vi "Compute Pseudo USC v2.vi"(4 "SDV (s)":dbl=160.0, 6 "Gaussian IRF":bool, 8 "Error In":errorcluster, 10 "Phasor Parameters":T2={"Display Parameters"={"# Points"=0, "Ramp Type"=enum."Linear", "Type of Series"=enum."1-Exp Decays", "Min tau"=0.0, "Max tau"=0.0, "Include 0"=FALSE, "Include Infinity"=FALSE}, "Phasor Parameters"={"Harmonic frequency"=0.0, "Use f* = 1/D Frequency"=FALSE, "Calibrated Phasor"=FALSE, "Calibration Lifetime"=1e-09, "Phasor Calculation"=enum."Direct Sum", "SEPL Type"=enum."UC", "# Gates"=1.0, "Square Gate Width"=1e-09, "Show Ticks"=FALSE}, "Decay & IRF Parameters"={"Lifetime"=0.0, "IRF Offset"=0.0, "Laser Period"=0.0, "Normalized Decays"=FALSE, "IRF Model"=enum."Dirac", "IRF Parameter 1"=0.0}, "Gate Parameters"={"First Gate Start"=0.0, "Use Gate Center"=FALSE, "Gate Width"=0.0, "Gate Step"=0.0, "# Gates"=0.0, "Gate Type"=enum."Square", "Edge Width"=0.0, "Top Slope"=0.0, "Reversed Sawtooth?"=FALSE, "Analytical Computation"=FALSE, "Tolerance"=1.0, "Integration"=enum."Item 0", "# Steps"=1.0, "Type of User-defined Function"=enum."Gate"}, "Detector Parameters"={"Frames/Image"=0, "Gates/Frame"=0, "Bits/Frame"=0, "Multiplicity"=0, "Incident Signal"=0.0}} {"Detector Parameters"."Frames/Image" min=1; "Detector Parameters"."Multiplicity" min=0; "Detector Parameters"."Bits/Frame" min=1; "Detector Parameters"."Gates/Frame" min=1; "Gate Parameters"."# Steps" min=0.0; "Gate Parameters"."Tolerance" min=0.0; "Gate Parameters"."Top Slope" min=0.0; "Gate Parameters"."Edge Width" min=0.0; "Gate Parameters"."Gate Step" min=0.0; "Gate Parameters"."# Gates" min=0.0 step=1.0; "Gate Parameters"."Gate Width" min=0.0; "Decay & IRF Parameters"."Lifetime" min=0.0; "Decay & IRF Parameters"."Laser Period" min=0.0; "Phasor Parameters"."Square Gate Width" min=0.0; "Phasor Parameters"."# Gates" min=0.0; "Phasor Parameters"."Calibration Lifetime" min=0.0; "Phasor Parameters"."Harmonic frequency" min=0.0; "Display Parameters"."Min tau" min=0.0; "Display Parameters"."Max tau" min=0.0; "Display Parameters"."# Points" min=1 step=1}, 11 "Phasor Graph Refnum":refnum<vi>) -> (0 "Error Out":errorcluster, 1 "Plot Name":string, 2 "Lifetime/Fraction Array":dbl[](array[numeric]), 3 "Single Exponential Phasor Plot":cluster{"Array":dbl[], "Array":dbl[]}, 5 "Phasor Calculation":T6, 7 "CPU (s)":dbl)   [LabVIEW 2019]
uses:
  Pseudo Phasor Parameters.ctl
  Phasor Explorer Display Parameters.ctl
  Type of Series.ctl
  Phasor Explorer Phasor Parameters.ctl
  Phasor Calculation Type.ctl
  Phasor Type.ctl
  Phasor Explorer Decay Parameters.ctl
  IRF Model.ctl
  Phasor Explorer Gate Parameters.ctl
  Gate Type.ctl
  Phasor Explorer Detector Parameters.ctl
  SEPXP Phasor Plot Info.ctl
  Phasor Calibration Data.ctl
  Phasor UC_N[W] Parameters.ctl
  <vilib>/Utility/High Resolution Relative Seconds.vi
panel:
  out "Plot Metadata":T1={"Lifetime/Fraction Array"=[], "Phasor Explorer Parameters"={"Display Parameters"={"# Points"=0, "Ramp Type"=enum."Linear", "Type of Series"=enum."1-Exp Decays", "Min tau"=0.0, "Max tau"=0.0, "Include 0"=FALSE, "Include Infinity"=FALSE}, "Phasor Parameters"={"Harmonic frequency"=0.0, "Use f* = 1/D Frequency"=FALSE, "Calibrated Phasor"=FALSE, "Calibration Lifetime"=1e-09, "Phasor Calculation"=enum."Direct Sum", "SEPL Type"=enum."UC", "# Gates"=1.0, "Square Gate Width"=1e-09, "Show Ticks"=FALSE}, "Decay & IRF Parameters"={"Lifetime"=0.0, "IRF Offset"=0.0, "Laser Period"=0.0, "Normalized Decays"=FALSE, "IRF Model"=enum."Dirac", "IRF Parameter 1"=0.0}, "Gate Parameters"={"First Gate Start"=0.0, "Use Gate Center"=FALSE, "Gate Width"=0.0, "Gate Step"=0.0, "# Gates"=0.0, "Gate Type"=enum."Square", "Edge Width"=0.0, "Top Slope"=0.0, "Reversed Sawtooth?"=FALSE, "Analytical Computation"=FALSE, "Tolerance"=1.0, "Integration"=enum."Item 0", "# Steps"=1.0, "Type of User-defined Function"=enum."Gate"}, "Detector Parameters"={"Frames/Image"=0, "Gates/Frame"=0, "Bits/Frame"=0, "Multiplicity"=0, "Incident Signal"=0.0}}, "Phase Lifetimes"=[], "Modulus Lifetimes"=[]} {"Phasor Explorer Parameters"."Detector Parameters"."Frames/Image" min=1; "Phasor Explorer Parameters"."Detector Parameters"."Multiplicity" min=0; "Phasor Explorer Parameters"."Detector Parameters"."Bits/Frame" min=1; "Phasor Explorer Parameters"."Detector Parameters"."Gates/Frame" min=1; "Phasor Explorer Parameters"."Gate Parameters"."# Steps" min=0.0; "Phasor Explorer Parameters"."Gate Parameters"."Tolerance" min=0.0; "Phasor Explorer Parameters"."Gate Parameters"."Top Slope" min=0.0; "Phasor Explorer Parameters"."Gate Parameters"."Edge Width" min=0.0; "Phasor Explorer Parameters"."Gate Parameters"."Gate Step" min=0.0; "Phasor Explorer Parameters"."Gate Parameters"."# Gates" min=0.0 step=1.0; "Phasor Explorer Parameters"."Gate Parameters"."Gate Width" min=0.0; "Phasor Explorer Parameters"."Decay & IRF Parameters"."Lifetime" min=0.0; "Phasor Explorer Parameters"."Decay & IRF Parameters"."Laser Period" min=0.0; "Phasor Explorer Parameters"."Phasor Parameters"."Square Gate Width" min=0.0; "Phasor Explorer Parameters"."Phasor Parameters"."# Gates" min=0.0; "Phasor Explorer Parameters"."Phasor Parameters"."Calibration Lifetime" min=0.0; "Phasor Explorer Parameters"."Phasor Parameters"."Harmonic frequency" min=0.0; "Phasor Explorer Parameters"."Display Parameters"."Min tau" min=0.0; "Phasor Explorer Parameters"."Display Parameters"."Max tau" min=0.0; "Phasor Explorer Parameters"."Display Parameters"."# Points" min=1 step=1}
  out "# Rejected Pairs":i32
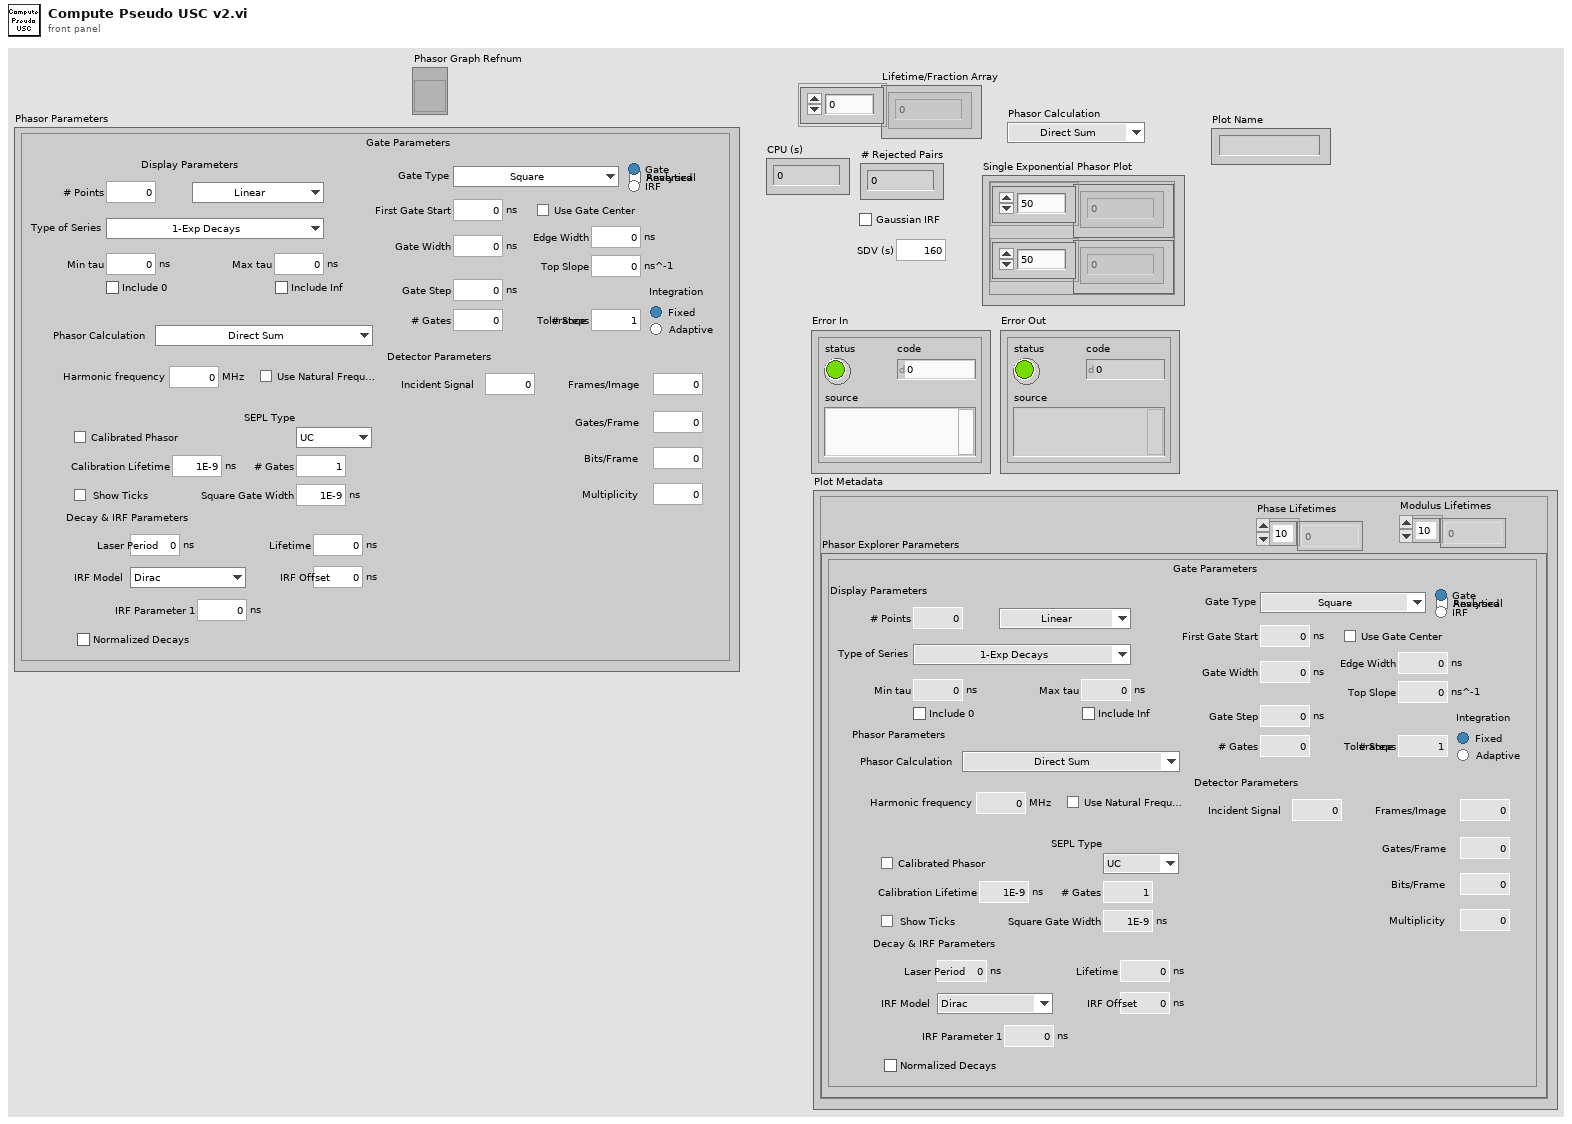
[diagram p1: front panel]
types:
  T1 = typedef "SEPXP Phasor Plot Info.ctl" = cluster{"Lifetime/Fraction Array":dbl[], "Phasor Explorer Parameters":T2, "Phase Lifetimes":dbl[], "Modulus Lifetimes":dbl[]}
  T2 = typedef "Pseudo Phasor Parameters.ctl" = cluster{"Display Parameters":T3, "Phasor Parameters":T5, "Decay & IRF Parameters":T8, "Gate Parameters":T10, "Detector Parameters":T12}
  T3 = typedef "Phasor Explorer Display Parameters.ctl" = cluster{"# Points":i32, "Ramp Type":enum16{"Linear", "Logarithmic"}, "Type of Series":T4, "Min tau":dbl[unit], "Max tau":dbl[unit], "Include 0":bool, "Include Infinity":bool}
  T4 = typedef "Type of Series.ctl" = enum16{"1-Exp Decays", "Linear Combination of 1-Exp"}
  T5 = typedef "Phasor Explorer Phasor Parameters.ctl" = cluster{"Harmonic frequency":dbl[unit], "Use f* = 1/D Frequency":bool, "Calibrated Phasor":bool, "Calibration Lifetime":dbl[unit], "Phasor Calculation":T6, "SEPL Type":T7, "# Gates":dbl, "Square Gate Width":dbl[unit], "Show Ticks":bool}
  T6 = typedef "Phasor Calculation Type.ctl" = enum16{"Direct Sum", "Analytical Formula"}
  T7 = typedef "Phasor Type.ctl" = enum16{"UC", "L_N", "L_N[W]"}
  T8 = typedef "Phasor Explorer Decay Parameters.ctl" = cluster{"Lifetime":dbl[unit], "IRF Offset":dbl[unit], "Laser Period":dbl[unit], "Normalized Decays":bool, "IRF Model":T9, "IRF Parameter 1":dbl[unit]}
  T9 = typedef "IRF Model.ctl" = enum16{"Dirac", "Exponential"}
  T10 = typedef "Phasor Explorer Gate Parameters.ctl" = cluster{"First Gate Start":dbl[unit], "Use Gate Center":bool, "Gate Width":dbl[unit], "Gate Step":dbl[unit], "# Gates":dbl, "Gate Type":T11, "Edge Width":dbl[unit], "Top Slope":dbl[unit], "Reversed Sawtooth?":bool, "Analytical Computation":bool, "Tolerance":dbl, "Integration":enum32{"Item 0", "Item 1"}, "# Steps":dbl, "Type of User-defined Function":enum32{"Gate", "IRF"}}
  T11 = typedef "Gate Type.ctl" = enum16{"Square", "Finite Edge Square", "Finite Edge, Tilted Top Square", "Triangle", "Sawtooth", "User-defined"}
  T12 = typedef "Phasor Explorer Detector Parameters.ctl" = cluster{"Frames/Image":i32, "Gates/Frame":i32, "Bits/Frame":i32, "Multiplicity":i32, "Incident Signal":dbl}
  T13 = typedef "Phasor UC_N[W] Parameters.ctl" = cluster{"Laser Period":dbl[unit], "Gate Width":dbl[unit], "Gate Step":dbl[unit], "Harmonic frequency":dbl[unit], "IRF offset":dbl[unit], "# Gates":dbl}
  T14 = typedef "Phasor Calibration Data.ctl" = cluster{"jw":cxt, "Uncalibrated Phasor":cxt, "Calibrated Phasor":cxt, "Calibrated Phasor?":bool, "Calibration Lifetime":ext}
  T15 = typedef "Gate Definitions.ctl" = cluster{"First Gate: t1":ext, "Gate Width: W":ext, "Gate Step: d":ext, "# Gates: G":ext, "Use Gate Center":bool, "Frames/Image: F":i32, "Gates/Frame: L":i32, "Bits/Frame: q":i32, "Multiplicity: p":i32, "Gate Type":T11, "Gate Edge s":ext, "Gate Top Slope":ext, "Reversed Sawtooth?":bool, "Computation":bool, "User-defined Gate":T16, "Tolerance":ext, "Integration":enum32{"Item 0", "Item 1"}, "# Steps":ext, "Type of User-defined Function":enum32{"Gate", "IRF"}}
  T16 = typedef "XY Plot Data.ctl" = cluster{"X Array":dbl[], "Y Array":dbl[]}
  T17 = typedef "Decay Definiton.ctl" = cluster{"offset: t0":ext, "period: T":ext, "lifetime: tau":ext, "Incident Signal: I":ext, "Normalized Decays":bool, "IRF Model":T9, "IRF Parameter 1":ext}
  T18 = cluster{"Numeric Control":ext, "Numeric Control":ext}
  T19 = cluster{"Calibrated g Array out":ext[], "Calibrated s Array out":ext[]}
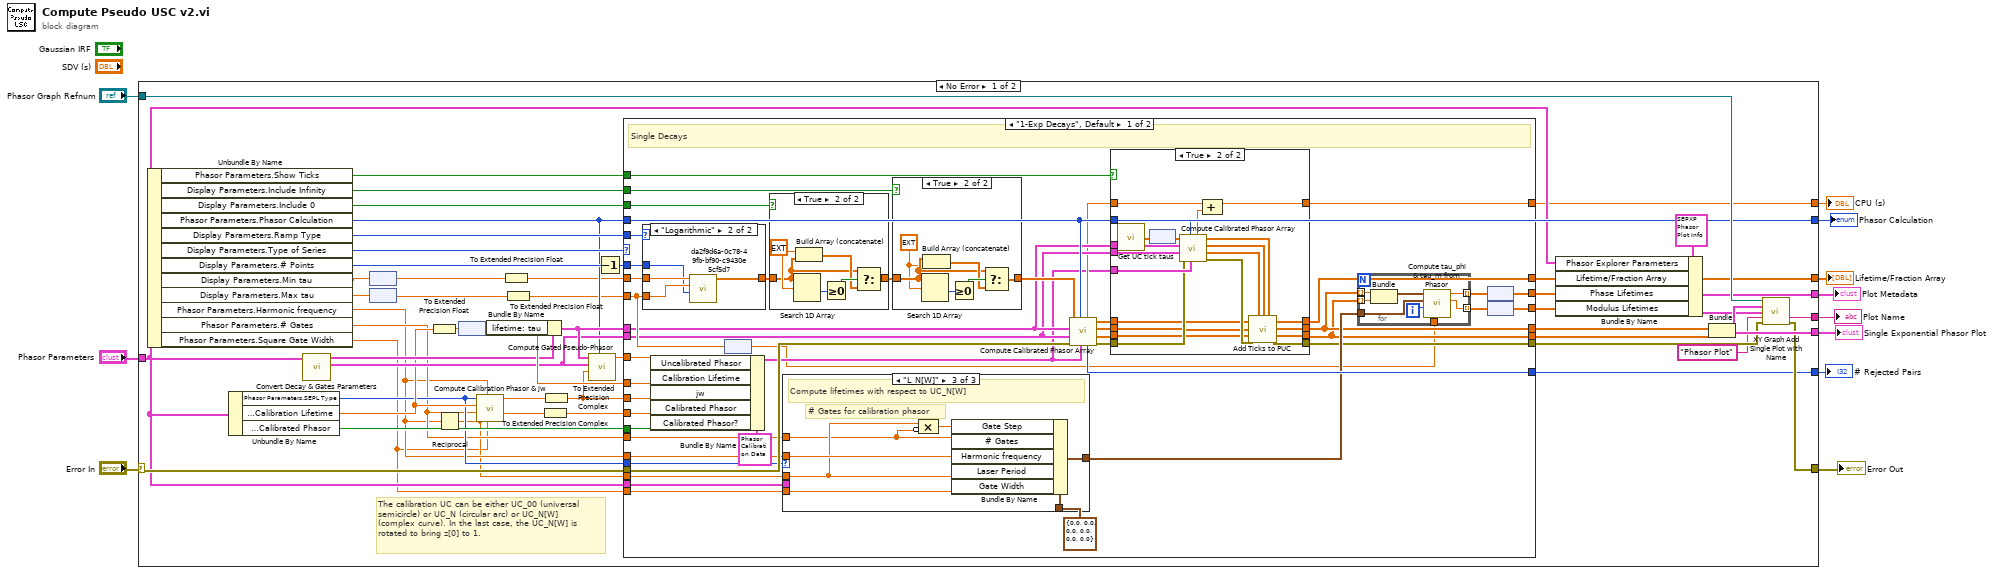
[diagram p0: block diagram]
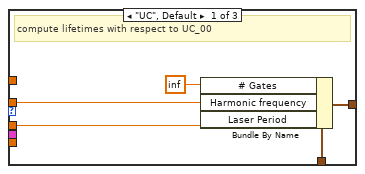
[diagram p3: hidden frame]
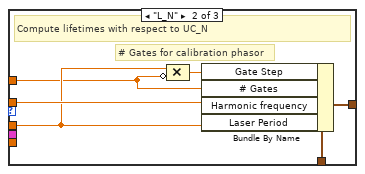
[diagram p4: hidden frame]
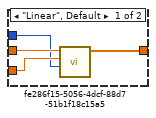
[diagram p7: hidden frame]
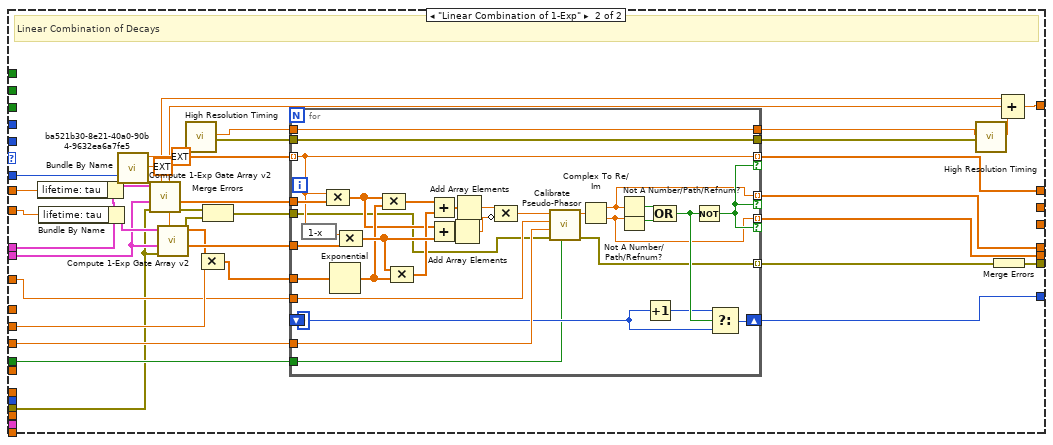
[diagram p8: hidden frame]
diagram:
  n1 = case shown="No Error" "Error In" {
    selector: "Error In" -> [w38 w248]
    tunnel: "Phasor Parameters" -> [w23 _]
    tunnel: [w52 _] -> w10
    tunnel: "Phasor Graph Refnum" -> [w53 _]
    tunnel: [w51 w248] -> w7
    tunnel: [w25 _] -> w6
    tunnel: [w39 _] -> w5
    tunnel: [w36 _] -> w4
    tunnel: [w31 _] -> w3
    tunnel: [w15 _] -> w2
    tunnel: [w12 _] -> w1
    frame No Error {
      # "The calibration UC can be either UC_00 (universal semicircle) or UC_N (circular arc) or UC_N[W] (complex curve). In the last case, the UC_N[W] is rotated to bring z[0] to 1."
      n2 = Unbundle By Name(w23) -> ("Phasor Parameters.Show Ticks"=w13:bool, "Display Parameters.Include Infinity"=w34:bool, "Display Parameters.Include 0"=w35:bool, "Phasor Parameters.Phasor Calculation"=w39:T6, "Display Parameters.Ramp Type"=w50:enum16{"Linear", "Logarithmic"}, "Display Parameters.Type of Series"=w43:T4, "Display Parameters.# Points"=w44:i32, "Display Parameters.Min tau"=w54:dbl[unit], "Display Parameters.Max tau"=w59:dbl[unit], "Phasor Parameters.Harmonic frequency"=w17:dbl[unit], "Phasor Parameters.# Gates"=w18:dbl, "Phasor Parameters.Square Gate Width"=w14:dbl[unit])
      n3 = Unbundle By Name(w23) -> ("Phasor Parameters.SEPL Type"=w19:T7, "Phasor Parameters.Calibration Lifetime"=w27:dbl[unit], "Phasor Parameters.Calibrated Phasor"=w40:bool)
      n4 = call "Convert Decay & Gates Parameters.vi"("Phasor Parameters"=w23) -> ("Gates Definitions"=w41:T15, "Decay Definition"=w42:T17)  [unwired: 9 in]
      n5 = node(w54) -> (w46:dbl)
      n6 = node(w59) -> (w45:dbl)
      n7 = To Extended Precision Float(1:w27) -> (0:w29:ext[unit])
      n8 = Reciprocal(x=w17) -> (1/x=w16:dbl[unit])
      n9 = node(w29) -> (w48:ext)
      n10 = call "Compute Calibration Phasor & jw.vi"("Gate Width"=w14, "Harmonic frequency"=w17, "Laser Period"=w16, "# Gates"=w18, "Calibration Lifetime"=w27, "Calibration Phasor Type"=w19) -> ("z (tau_cal)"=w20:cdb, "i 2 pi f (GHz)"=w47:cdb)  [unwired: 4 in]
      n11 = Bundle By Name(cluster=w42, "lifetime: tau"=w48) -> (w55:T17)
      n12 = To Extended Precision Float(1:w46) -> (0:w33:ext)
      n13 = To Extended Precision Float(1:w45) -> (0:w32:ext)
      n14 = To Extended Precision Complex(1:w20) -> (0:w30:cxt)
      n15 = To Extended Precision Complex(1:w47) -> (0:w28:cxt)
      n16 = call "Compute Gated Pseudo-Phasor.vi"("Phasor Calculation Type"=w39, "j 2 pi f"=w28, "Gates Definitions"=w41, "Decay Definition"=w55) -> ("phasor"=w56:cxt)  [unwired: 5 in, 2 out]
      n17 = Decrement(x=w44) -> (x-1=w49:i32)
      n18 = case shown="\"1-Exp Decays\", Default" w43 {
        tunnel: [w62 w192] -> w58
        tunnel: [w61 w191] -> w57
        tunnel: w40 -> [w98 w201]
        tunnel: w56 -> [w101 w199]
        tunnel: w55 -> [w73 w214]
        tunnel: w41 -> [w72 w210]
        tunnel: w28 -> [w97 w203]
        tunnel: w30 -> [w100 w200]
        tunnel: w33 -> [w104 w215]
        tunnel: w32 -> [w76 w213]
        tunnel: w49 -> [w103 w207]
        tunnel: w50 -> [w102 _]
        tunnel: w48 -> [w96 _]
        tunnel: w39 -> [w75 _]
        tunnel: [w63 w193] -> w25
        tunnel: w38 -> [w95 w198]
        tunnel: [w71 w179] -> w37
        tunnel: w35 -> [w93 _]
        tunnel: w34 -> [w91 _]
        tunnel: [w89 w194] -> w31
        tunnel: w23 -> [w88 _]
        tunnel: [w84 _] -> w22
        tunnel: [w85 _] -> w21
        tunnel: w19 -> [w82 _]
        tunnel: w17 -> [w80 _]
        tunnel: w16 -> [w79 _]
        tunnel: w18 -> [w78 _]
        tunnel: [w69 w184] -> w15
        tunnel: w14 -> [w77 _]
        tunnel: w13 -> [w74 _]
        frame "1-Exp Decays", Default {
          # "Single Decays"
          n19 = case shown="\"Logarithmic\"" w102 {
            tunnel: w104 -> [w174 w177]
            tunnel: w76 -> [w173 w176]
            tunnel: w103 -> [w172 w175]
            tunnel: [w171 w178] -> w94
            frame "Linear", Default {
              n20 = call "fe286f15-5056-4dcf-88d7-51b1f18c15a5.vi"("# Steps (1)"=w172, "End (1)"=w173, "Start (0)"=w174) -> ("Ramp"=w171:ext[])  [unwired: 7 in, 1 out]
            }
            frame "Logarithmic" {
              n21 = call "da2f9d6a-0c78-49fb-bf90-c9430e5cf5d7.vi"("# Steps (1)"=w175, "End (1)"=w176, "Start (1)"=w177) -> ("Ramp"=w178:ext[])  [unwired: 7 in, 1 out]
            }
          }
          n22 = Bundle By Name(cluster=T14 {"jw"=0.0+0.0i, "Uncalibrated Phasor"=0.0+0.0i, "Calibrated Phasor"=0.0+0.0i, "Calibrated Phasor?"=FALSE, "Calibration Lifetime"=0.0} ("output cluster"), "Uncalibrated Phasor"=w101, "Calibration Lifetime"=w96, "jw"=w97, "Calibrated Phasor"=w100, "Calibrated Phasor?"=w98) -> (w65:T14)
          n23 = node(w76) -> (w60:ext[unit])
          n24 = case shown="True" w93 {
            tunnel: w94 -> [w164 w166]
            tunnel: [w164 w165] -> w92
            frame False {
            }
            frame True {
              w168 = ext 0.0 ("element")
              n25 = Search 1D Array(1D array=w166, element=w168) -> (index of element=w170:i32)  [unwired: 1 in]
              n26 = Build Array (concatenate)(w168, w166) -> (w167:ext[])
              n27 = Greater Or Equal To 0?(x=w170) -> (x >= 0?=w169:bool)
              n28 = Select(t=w166, s=w169, f=w167) -> (s? t:f=w165:ext[])
            }
          }
          n29 = case shown="\"L_N[W]\"" w82 {
            tunnel: w88 -> [_ _ _]
            tunnel: [w135 w141 w148] -> w83
            tunnel: T13 {"Laser Period"=0.0, "Gate Width"=0.0, "Gate Step"=0.0, "Harmonic frequency"=0.0, "IRF offset"=0.0, "# Gates"=0.0} ("Phasor UCN[W] Parameters") -> [w133 w140 w147]
            tunnel: w80 -> [w132 w139 w146]
            tunnel: w79 -> [w131 w138 w145]
            tunnel: w78 -> [_ w136 w143]
            tunnel: w77 -> [_ _ w142]
            frame "UC", Default {
              # "compute lifetimes with respect to UC_00"
              n30 = Bundle By Name(cluster=w133, "# Gates"=inf ("Gate Parameters.# Gates"), "Harmonic frequency"=w132, "Laser Period"=w131) -> (w135:T13)
            }
            frame "L_N" {
              # "# Gates for calibration phasor"
              # "Compute lifetimes with respect to UC_N"
              n31 = Compound Arithmetic op=MULTIPLY(w138, invert w136) -> (w137:dbl[unit])
              n32 = Bundle By Name(cluster=w140, "Gate Step"=w137, "# Gates"=w136, "Harmonic frequency"=w139, "Laser Period"=w138) -> (w141:T13)
            }
            frame "L_N[W]" {
              # "# Gates for calibration phasor"
              # "Compute lifetimes with respect to UC_N[W]"
              n33 = Compound Arithmetic op=MULTIPLY(w145, invert w143) -> (w144:dbl[unit])
              n34 = Bundle By Name(cluster=w147, "Gate Step"=w144, "# Gates"=w143, "Harmonic frequency"=w146, "Laser Period"=w145, "Gate Width"=w142) -> (w148:T13)
            }
          }
          n35 = case shown="True" w91 {
            tunnel: w92 -> [w157 w160]
            tunnel: [w157 w159] -> w90
            frame False {
            }
            frame True {
              w158 = ext inf ("element")
              n36 = Search 1D Array(1D array=w160, element=w158) -> (index of element=w163:i32)  [unwired: 1 in]
              n37 = Build Array (concatenate)(w160, w158) -> (w161:ext[])
              n38 = Greater Or Equal To 0?(x=w163) -> (x >= 0?=w162:bool)
              n39 = Select(t=w160, s=w162, f=w161) -> (s? t:f=w159:ext[])
            }
          }
          n40 = call "Compute Calibrated Phasor Array.vi"("Phasor Calibration Data"=w65, "Phasor Calculation"=w75, "Error In"=w95, "Gates Definitions"=w72, "Decay Definition"=w73, "Lifetime Array"=w90) -> ("Error Out"=w64:errorcluster, "Calibrated s Array"=w66:ext[], "Calibrated g Array"=w67:ext[], "True Lifetime Array"=w68:ext[], "# Rejected Pairs"=w89:i32, "CPU (s)"=w70:dbl)
          n41 = case shown="True" w74 {
            tunnel: w75 -> [_ w130]
            tunnel: w73 -> [_ w129]
            tunnel: w72 -> [_ w128]
            tunnel: [w108 w119] -> w71
            tunnel: w70 -> [w109 w127]
            tunnel: [w109 w125] -> w69
            tunnel: w68 -> [w107 w117]
            tunnel: w67 -> [w106 w116]
            tunnel: w66 -> [w105 w115]
            tunnel: w65 -> [_ w122]
            tunnel: w64 -> [w108 w121]
            tunnel: [w107 w114] -> w63
            tunnel: [w106 w113] -> w62
            tunnel: [w105 w112] -> w61
            frame False {
            }
            frame True {
              n42 = call "Get UC tick taus.vi"() -> ("Array of taus"=w124:dbl[unit][])  [unwired: 8 in]
              n43 = node(w124) -> (w123:dbl[])
              n44 = call "Compute Calibrated Phasor Array.vi"("Phasor Calibration Data"=w122, "Phasor Calculation"=w130, "Error In"=w121, "Gates Definitions"=w128, "Decay Definition"=w129, "Lifetime Array"=w123) -> ("Error Out"=w120:errorcluster, "Calibrated s Array"=w111:ext[], "Calibrated g Array"=w110:ext[], "True Lifetime Array"=w118:ext[], "CPU (s)"=w126:dbl)  [unwired: 1 out]
              n45 = Compound Arithmetic op=ADD(w127, w126) -> (w125:dbl)
              n46 = call "Add Ticks to PUC.vi"("Ticks Calibrated s's"=w111, "Ticks Calibrated g's"=w110, "Ticks Lifetimes"=w118, "Lifetime Array in"=w117, "Calibrated g Array in"=w116, "Calibrated s Array in"=w115, "error in (no error)"=w120) -> ("Lifetime Array out"=w114:ext[], "Calibrated g Array out"=w113:ext[], "Calibrated s Array out"=w112:ext[], "error out"=w119:errorcluster)  [unwired: 5 in]
            }
          }
          n47 = for {
            tunnel: w60 -> [w150]
            tunnel: w83 -> [w151]
            tunnel: w62 -> [w154] mode=indexing
            tunnel: w61 -> [w153] mode=indexing
            tunnel: [w156] -> w87 mode=indexing
            tunnel: [w155] -> w86 mode=indexing
            i -> [w149]
            n48 = Bundle("Numeric Control"=w154, "Numeric Control"=w153) -> (w152:T18)  [unwired: 1 in]
            n49 = call "Compute tau_phi & tau_m from Phasor.vi"("max tau"=w150, "Call # (0)"=w149, "Phasor UCN[W] Parameters"=w151, "Phasor"=w152) -> ("tau_m"=w156:dbl[unit], "tau_ph"=w155:dbl[unit])  [unwired: 5 in, 1 out]
          }
          n50 = node(w86) -> (w85:dbl[])
          n51 = node(w87) -> (w84:dbl[])
        }
        frame "Linear Combination of 1-Exp" {
          # "Linear Combination of Decays"
          n52 = Bundle By Name(cluster=w214, "lifetime: tau"=w215) -> (w212:T17)
          n53 = Bundle By Name(cluster=w214, "lifetime: tau"=w213) -> (w211:T17)
          n54 = call "ba521b30-8e21-40a0-90b4-9632ea6a7fe5.vi"("# Steps (1)"=w207, "End (1)"=ext 1.0 ("Max"), "Start (0)"=ext 0.0 ("Min")) -> ("Ramp"=w195:ext[])  [unwired: 7 in, 1 out]
          n55 = call "Compute 1-Exp Gate Array v2.vi"("Error In"=w198, "Gates Definitions"=w210, "Decay Definition"=w212) -> ("Error Out"=w197:errorcluster, "Gate Image Array"=w206:ext[], "CPU (s)"=w183:dbl)  [unwired: 4 in, 2 out]
          n56 = call "Compute 1-Exp Gate Array v2.vi"("Error In"=w198, "Gates Definitions"=w210, "Decay Definition"=w211) -> ("Error Out"=w196:errorcluster, "Gate Image Array"=w205:ext[], "t Array"=w204:ext[], "CPU (s)"=w182:dbl)  [unwired: 4 in, 1 out]
          n57 = call "High Resolution Timing.vi"() -> ("elapsed (relative) seconds"=w187:dbl, "Error Out"=w189:errorcluster)  [unwired: 17 in, 1 out]
          n58 = Compound Arithmetic op=MULTIPLY(w204, w203) -> (w202:cxt[])
          n59 = Merge Errors(w197, w196) -> (w181:errorcluster)
          n60 = for {
            tunnel: w206 -> [w247]
            tunnel: w205 -> [w246]
            tunnel: w195 -> [w227] mode=indexing
            tunnel: w202 -> [w245]
            tunnel: [w223] -> w191 mode=indexing if=w226
            tunnel: [w222] -> w192 mode=indexing if=w226
            tunnel: w201 -> [w218]
            tunnel: w200 -> [w232]
            tunnel: w199 -> [w231]
            tunnel: [w227] -> w193 mode=indexing if=w226
            shift-right: [w225] -> w194
            shift-left: 0 -> [w224]
            tunnel: w189 -> [w220]
            tunnel: [w220] -> w188
            tunnel: w187 -> [w219]
            tunnel: [w219] -> w186
            tunnel: w181 -> [w217]
            tunnel: [w216] -> w180 mode=indexing
            n61 = expression code="1-x"(w227) -> (w242:ext)
            n62 = Compound Arithmetic op=MULTIPLY(w227, w247) -> (w237:ext[])
            n63 = Exponential(1:w245) -> (0:w243:cxt[])
            n64 = Compound Arithmetic op=MULTIPLY(w242, w246) -> (w244:ext[])
            n65 = Compound Arithmetic op=MULTIPLY(w237, w243) -> (w241:cxt[])
            n66 = Compound Arithmetic op=MULTIPLY(w244, w243) -> (w240:cxt[])
            n67 = Add(x=w241, y=w240) -> (x+y=w239:cxt[])
            n68 = Add(x=w237, y=w244) -> (x+y=w238:ext[])
            n69 = Add Array Elements(numeric array=w238) -> (sum=w235:ext)
            n70 = Add Array Elements(numeric array=w239) -> (sum=w236:cxt)
            n71 = Compound Arithmetic op=MULTIPLY(w236, invert w235) -> (w234:cxt)
            n72 = call "Calibrate Pseudo-Phasor.vi"("Calibrated Phasor"=w218, "Error In"=w217, "Target Phasor"=w232, "Calibration Pseudo-Phasor"=w231, "Pseudo-Phasor in"=w234) -> ("Error Out"=w216:errorcluster, "Pseudo-Phasor out"=w233:cxt)  [unwired: 5 in]
            n73 = Complex To Re/Im(x + iy=w233) -> (x=w222:ext, y=w223:ext)
            n74 = Not A Number/Path/Refnum?(number/path/refnum=w222) -> (NaN/Path/Refnum?=w221:bool)
            n75 = Not A Number/Path/Refnum?(number/path/refnum=w223) -> (NaN/Path/Refnum?=w230:bool)
            n76 = Increment(x=w224) -> (x+1=w228:i32)
            n77 = Compound Arithmetic op=OR(w221, w230) -> (w229:bool)
            n78 = Not(x=w229) -> (.not. x?=w226:bool)
            n79 = Select(t=w228, s=w229, f=w224) -> (s? t:f=w225:i32)
          }
          n80 = call "High Resolution Timing.vi"("relative seconds (NaN)"=w186, "Error In"=w188) -> ("elapsed (relative) seconds"=w185:dbl)  [unwired: 15 in, 2 out]
          n81 = Merge Errors(w180) -> (w179:errorcluster)
          n82 = Compound Arithmetic op=ADD(w183, w182, w185) -> (w184:dbl)
        }
      }
      n83 = Bundle By Name(cluster=T1 {"Lifetime/Fraction Array"=[], "Phasor Explorer Parameters"={"Display Parameters"={"# Points"=0, "Ramp Type"=enum."Linear", "Type of Series"=enum."1-Exp Decays", "Min tau"=0.0, "Max tau"=0.0, "Include 0"=FALSE, "Include Infinity"=FALSE}, "Phasor Parameters"={"Harmonic frequency"=0.0, "Use f* = 1/D Frequency"=FALSE, "Calibrated Phasor"=FALSE, "Calibration Lifetime"=1e-09, "Phasor Calculation"=enum."Direct Sum", "SEPL Type"=enum."UC", "# Gates"=1.0, "Square Gate Width"=1e-09, "Show Ticks"=FALSE}, "Decay & IRF Parameters"={"Lifetime"=0.0, "IRF Offset"=0.0, "Laser Period"=0.0, "Normalized Decays"=FALSE, "IRF Model"=enum."Dirac", "IRF Parameter 1"=0.0}, "Gate Parameters"={"First Gate Start"=0.0, "Use Gate Center"=FALSE, "Gate Width"=0.0, "Gate Step"=0.0, "# Gates"=0.0, "Gate Type"=enum."Square", "Edge Width"=0.0, "Top Slope"=0.0, "Reversed Sawtooth?"=FALSE, "Analytical Computation"=FALSE, "Tolerance"=1.0, "Integration"=enum."Item 0", "# Steps"=1.0, "Type of User-defined Function"=enum."Gate"}, "Detector Parameters"={"Frames/Image"=0, "Gates/Frame"=0, "Bits/Frame"=0, "Multiplicity"=0, "Incident Signal"=0.0}}, "Phase Lifetimes"=[], "Modulus Lifetimes"=[]} ("Phasor Graph Plot Info"), "Phasor Explorer Parameters"=w23, "Lifetime/Fraction Array"=w25, "Phase Lifetimes"=w21, "Modulus Lifetimes"=w22) -> (w12:T1)
      n84 = Bundle("Calibrated g Array out"=w58, "Calibrated s Array out"=w57) -> (w52:T19)  [unwired: 1 in]
      n85 = call "XY Graph Add Single Plot with Name.vi"("XYGraph Ref in"=w53, "Plot"=w52, "Plot Metadata"=w12, "Plot Name (\"Plot\")"="Phasor Plot" ("Plot Name (\"Plot\")"), "error in (no error)"=w37) -> ("Plot Name"=w36:string, "error out"=w51:errorcluster)  [unwired: 7 in, 2 out]
    }
    frame Error {
    }
  }
  "Error Out" <- w7
  "Single Exponential Phasor Plot" <- w10
  "Lifetime/Fraction Array" <- w6
  "Phasor Calculation" <- w5
  "Plot Name" <- w4
  "# Rejected Pairs" <- w3
  "CPU (s)" <- w2
  "Plot Metadata" <- w1
